vi "initiate_mark_10.vi"(8 "error in":errorcluster, 11 "VISA Refnum in":refnum<visa-resource-name>) -> (0 "error out":errorcluster, 3 "VISA Refnum out":refnum<visa-resource-name>)   [LabVIEW 2017]
uses:
  serial_setting_1.ctl
  <vilib>/Instr/_visa.llb/VISA Configure Serial Port (Instr).vi
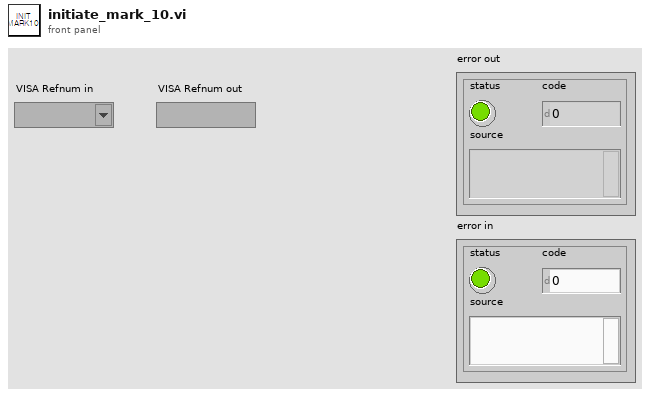
[diagram p1: front panel]
types:
  T1 = typedef "serial_setting_1.ctl" = cluster{"baud rate":u32, "data bits":u16, "parity":enum16{"None", "Odd", "Even", "Mark", "Space"}, "stop bits":u16, "flow control":u16, "IsConfigured":bool}
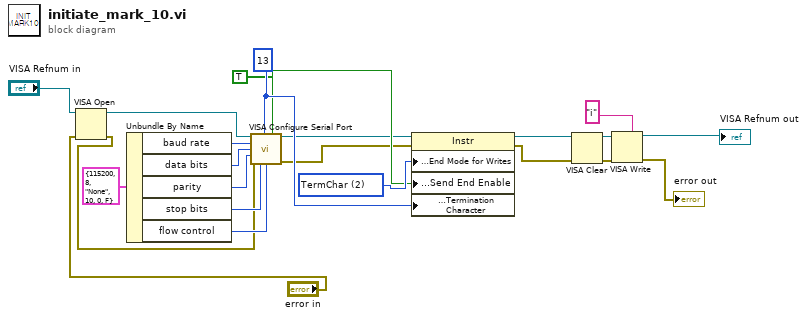
[diagram p0: block diagram]
diagram:
  w21 = u16 2 items=["None", "Last Bit", "TermChar", "Break"] ("Serial Settings:End Mode for Writes")
  w18 = TRUE
  w19 = u8 13 ("Termination Character")
  n1 = VISA Open(error in (no error)="error in", VISA resource name="VISA Refnum in") -> (VISA resource name=w5:refnum<visa-resource-name>, error out=w1:errorcluster)  [unwired: 3 in]
  n2 = Unbundle By Name(T1 {"baud rate"=115200, "data bits"=8, "parity"=enum."None", "stop bits"=10, "flow control"=0, "IsConfigured"=FALSE} ("Serial Settings")) -> ("baud rate"=w16:u32, "data bits"=w15:u16, "parity"=w14:enum16{"None", "Odd", "Even", "Mark", "Space"}, "stop bits"=w13:u16, "flow control"=w12:u16)
  n3 = call-poly "VISA Configure Serial Port"("VISA resource name"=w5, "termination char\n(0xA = '\\n' = LF)"=w19, "Enable Termination\nChar (T)"=w18, "baud rate (9600)"=w16, "data bits (8)"=w15, "parity (0:none)"=w14, "error in (no error)"=w1, "stop bits (10: 1 bit)"=w13, "flow control (0:none)"=w12) -> ("VISA resource name out"=w11:refnum<visa-resource-name>, "error out"=w10:errorcluster)  [unwired: 5 in]
  n4 = property class="Instr"(reference=w11, error in=w10, "Serial Settings:End Mode for Writes"=w21, "Message Based Settings:Send End Enable"=w18, "Message Based Settings:Termination Character"=w19) -> (reference out=w7:refnum<visa-resource-name>, error out=w6:errorcluster)
  n5 = VISA Clear(VISA resource name=w7, error in (no error)=w6) -> (VISA resource name out=w9:refnum<visa-resource-name>, error out=w8:errorcluster)
  n6 = VISA Write(VISA resource name=w9, write buffer="i", error in (no error)=w8) -> (VISA resource name out=→"VISA Refnum out":refnum<visa-resource-name>, error out=→"error out":errorcluster)  [unwired: 1 out]
